vi "get channels test.vi"() -> ()   [LabVIEW 2013, in "Shared Memory tests.lvlib"]
doc: "Tests the 'Get Channels' VI of the Configuration class."
uses:
  Shared Memory tests.lvlib
  module/configuration/Shared Memory configuration.lvclass
panel:
  out "error out":errorcluster
  out "channels match":bool
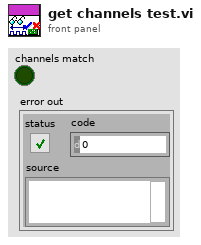
[diagram p1: front panel]
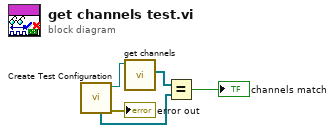
[diagram p0: block diagram]
diagram:
  n1 = call "Create Test Configuration.vi"() -> ("error out"=→"error out":errorcluster, "Module Configuration"=w3:refnum<class "Shared Memory configuration.lvclass">, "Channels"=w1:refnum<class "TBM channel.lvclass">[])  [unwired: 6 in, 3 out]
  n2 = call-dynamic "get channels.vi"("Shared Memory configuration in"=w3) -> ("channels"=w5:refnum<class "TBM channel.lvclass">[])  [unwired: 9 in, 1 out]
  n3 = Equal?(x=w5, y=w1) -> (x = y?=→"channels match":bool)
